vi "Write Requirements Path.vi"(10 "URI":string, 11 "Project in":refnum<class "RequirementMap.lvclass">) -> (3 "Project out":refnum<class "RequirementMap.lvclass">)   [LabVIEW 2021, in "Bananas.lvlib" / "RequirementMap.lvclass"]
uses:
  RequirementMap.lvclass
  RequirementMap.lvclass/RequirementMap.ctl
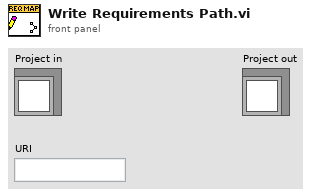
[diagram p1: front panel]
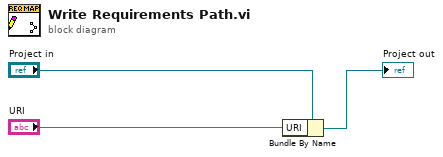
[diagram p0: block diagram]
diagram:
  n1 = Bundle By Name(cluster="Project in", "URI"="URI") -> (→"Project out":refnum<class "RequirementMap.lvclass">)
